vi "synth_set(SubVI).vi"(3 "dc offset?":bool=TRUE, 6 "error in (no error)":errorcluster, 7 "User Def. Wfm Name":string, 8 "chirp?":bool, 9 "VISA session":refnum<visa-resource-name>, 10 "amplitude (V)":ext=2.5, 11 "frequency (Hz)":ext=76.5) -> (2 "dup VISA session":refnum<visa-resource-name>, 4 "error out":errorcluster)   [LabVIEW 2012]
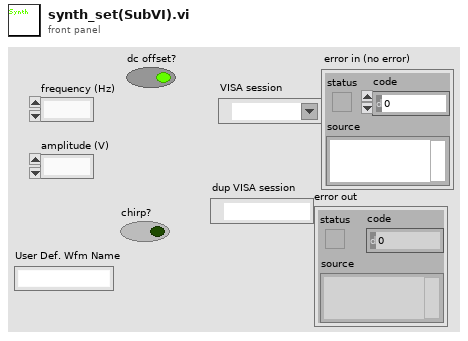
[diagram p1: front panel]
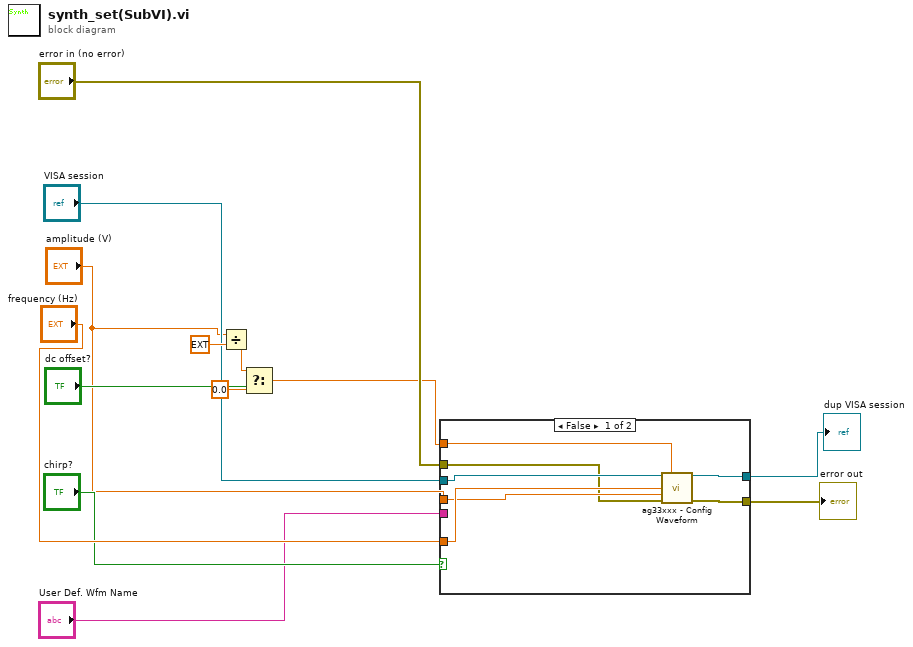
[diagram p0: block diagram]
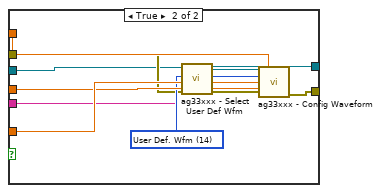
[diagram p2: hidden frame]
diagram:
  n1 = Divide(x="amplitude (V)", y=ext 2.0) -> (x/y=w11:ext)
  n2 = Select(t=w11, s="dc offset?", f=0.0) -> (s? t:f=w7:ext)
  n3 = case shown="False" "chirp?" {
    tunnel: "VISA session" -> [w15 w24]
    tunnel: "error in (no error)" -> [w14 w25]
    tunnel: w7 -> [w20 w31]
    tunnel: "frequency (Hz)" -> [w19 w30]
    tunnel: "amplitude (V)" -> [w18 w29]
    tunnel: [w17 w27] -> w4
    tunnel: [w16 w26] -> w3
    tunnel: "User Def. Wfm Name" -> [_ w21]
    frame False {
      n4 = call <vilib>:"ag33xxx - Config Waveform.vi"("VISA session"=w15, "Offset (0.00 V)"=w20, "Frequency (1000 Hz)"=w19, "Amplitude (0.1 Vpp)"=w18, "error in (no error)"=w14) -> ("dup VISA session"=w16:refnum<visa-resource-name>, "error out"=w17:errorcluster)  [unwired: 9 in]
    }
    frame True {
      w28 = u16 14 items=["DC"=0, "Sine"=1, "Square"=2, "Triangle"=3, "Ramp"=4, "Pulse"=6, "Noise"=7, "Sinc"=8, "Neg. Ramp"=9, "Exp. Rise"=10, "Exp. Fall"=11, "Cardiac"=12, "Volatile"=13, "User Def. Wfm"=14] ("Waveform Shape (1: Sine)")
      n5 = call <vilib>:"ag33xxx - Select User Def Wfm.vi"("error in (no error)"=w25, "User Def. Wfm Name"=w21, "VISA session"=w24) -> ("error out"=w22:errorcluster, "dup VISA session"=w23:refnum<visa-resource-name>)  [unwired: 7 in]
      n6 = call <vilib>:"ag33xxx - Config Waveform.vi"("VISA session"=w23, "Offset (0.00 V)"=w31, "Waveform Shape (1: Sine)"=w28, "Frequency (1000 Hz)"=w30, "Amplitude (0.1 Vpp)"=w29, "error in (no error)"=w22) -> ("dup VISA session"=w26:refnum<visa-resource-name>, "error out"=w27:errorcluster)  [unwired: 8 in]
    }
  }
  "error out" <- w4
  "dup VISA session" <- w3
